vi "pathfinder prepare.vi"(0 "path":T1[](array[typedef]), 1 "sample_count":i32=10000, 5 "max_velocity":dbl, 7 "max_acceleration":dbl, 9 "max_jerk":dbl, 11 "error in (no error)":errorcluster, 12 "dt":dbl) -> (4 "function return":i32, 15 "error out":errorcluster)   [LabVIEW 2017, in "Pathfinder.lvlib"]
doc: "CAPI int pathfinder_prepare_LabVIEW(const Waypoint *path, int path_length, int sample_count, double dt,\n double max_velocity, double max_acceleration, double max_jerk);"
uses:
  Pathfinder.lvlib
  Waypoint.ctl
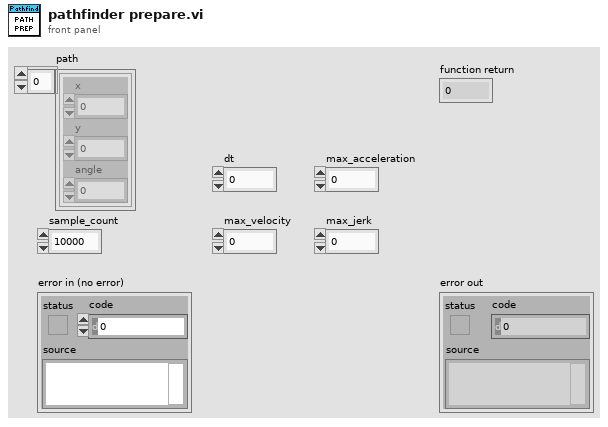
[diagram p1: front panel]
types:
  T1 = typedef "Pathfinder.lvlib/Waypoint.ctl" = cluster{"x":dbl, "y":dbl, "angle":dbl}
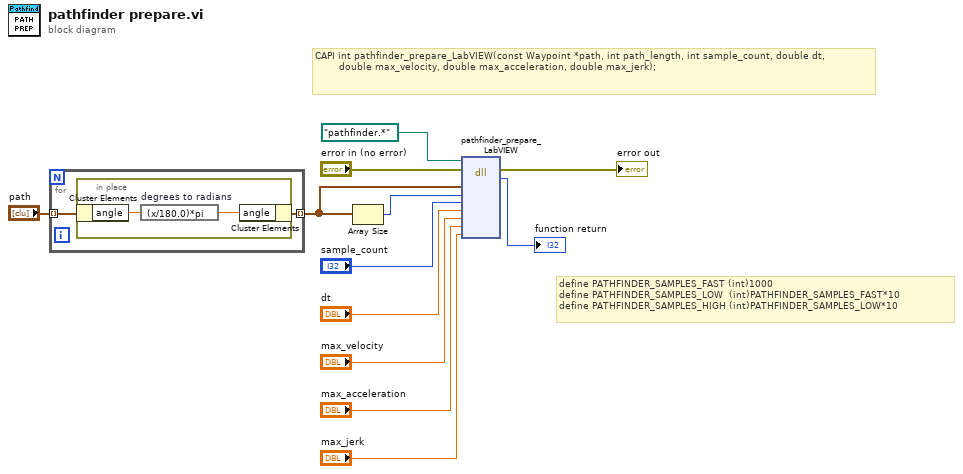
[diagram p0: block diagram]
diagram:
  # "define PATHFINDER_SAMPLES_FAST (int)1000\ndefine PATHFINDER_SAMPLES_LOW  (int)PATHFINDER_SAMPLES_FAST*10\ndefine PATHFINDER_SAMPLES_HIGH (int)PATHFINDER_SAMPLES_LOW*10"
  # "CAPI int pathfinder_prepare_LabVIEW(const Waypoint *path, int path_length, int sample_count, double dt,\n        double max_velocity, double max_acceleration, double max_jerk);"
  n1 = for {
    tunnel: "path" -> [w14] mode=indexing
    tunnel: [w13] -> w5 mode=indexing
    n2 = in-place {
      n3 = in-place-cluster #1(w14) -> ("angle"=w16:dbl)
      n4 = expression code="(x/180.0)*pi" "degrees to radians"(w16) -> (w15:dbl)
      n5 = in-place-cluster #1("angle"=w15) -> (w13:T1)
    }
  }
  n6 = Array Size(array=w5) -> (size(s)=w4:i32)
  n7 = dll-call lib="?" fn="pathfinder_prepare_LabVIEW"(path in=path "pathfinder.*", error in="error in (no error)", "path"=w5, "path_length"=w4, "sample_count"="sample_count", "dt"="dt", "max_velocity"="max_velocity", "max_acceleration"="max_acceleration", "max_jerk"="max_jerk") -> (error out=→"error out":errorcluster, "return type"=→"function return":i32)  [unwired: 8 in, 1 out]
